vi "Byte Buffer.Read (SGL).vi"(8 "error in (no error)":errorcluster, 10 "buffer offset":u64, 11 "Byte Buffer in":refnum<class "Byte Buffer.lvclass">) -> (0 "error out":errorcluster, 1 "value":sgl, 3 "Byte Buffer out":refnum<class "Byte Buffer.lvclass">)   [LabVIEW 2016, in "VeriStand Data.lvlib" / "Byte Buffer.lvclass"]
doc: "Reads one element of data from the provided <B>Byte Buffer</B> at location <B>buffer offset</B> in the format of the data type specified."
uses:
  Byte Buffer.lvclass
  Byte Buffer.lvclass/Byte Buffer.ctl
  Byte Buffer.Allocate.vi
  Byte Buffer.Get Buffer Subset.vi
  Memory Management/Memory Management.MoveByteBlock.Write (String).vi
  Memory Management/Memory Management.Handle Return.vi
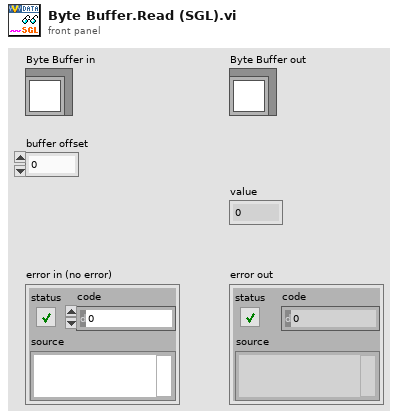
[diagram p1: front panel]
types:
  T1 = enum16{"big-endian, network order", "native, host order", "little-endian"}
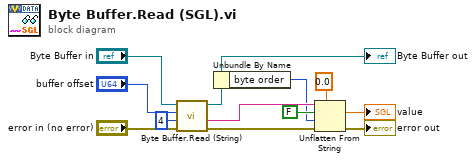
[diagram p0: block diagram]
diagram:
  n1 = call "Byte Buffer.Read (String).vi"("error in (no error)"="error in (no error)", "count"=i64 4, "buffer offset"="buffer offset", "Byte Buffer in"="Byte Buffer in") -> ("error out"=w6:errorcluster, "string"=w2:string, "Byte Buffer out"=w3:refnum<class "Byte Buffer.lvclass">)  [unwired: 5 in]
  "Byte Buffer out" <- w3
  n2 = Unbundle By Name(w3) -> ("byte order"=w1:T1)
  n3 = Unflatten From String(type=sgl 0.0 ("Boolean"), binary string=w2, data includes array or string size? (T)=FALSE, byte order (0:big-endian, network order)=w1, error in (no error)=w6) -> (value=→"value":sgl, error out=→"error out":errorcluster)  [unwired: 1 out]
